vi "FitEllipse2.vi"(6 "Reject Outliers":bool, 10 "Input data":cluster{"Numeric":dbl, "Numeric":dbl}[](array[cluster])) -> (1 "XY Fit":cluster{dbl[], dbl[]}, 3 "Ellipse":T1, 5 "Valid Fit":bool)   [LabVIEW 2011]
uses:
  <vilib>/vision/NI_Vision_Development_Module.lvlib
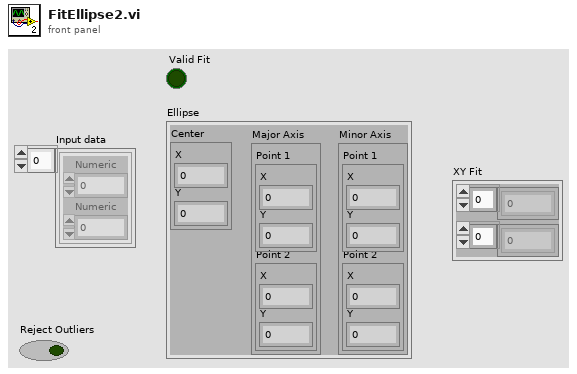
[diagram p1: front panel]
types:
  T1 = cluster{"Center":cluster{"X":sgl, "Y":sgl}, "Major Axis":cluster{"Point 1":cluster{"X":sgl, "Y":sgl}, "Point 2":cluster{"X":sgl, "Y":sgl}}, "Minor Axis":cluster{"Point 1":cluster{"X":sgl, "Y":sgl}, "Point 2":cluster{"X":sgl, "Y":sgl}}}
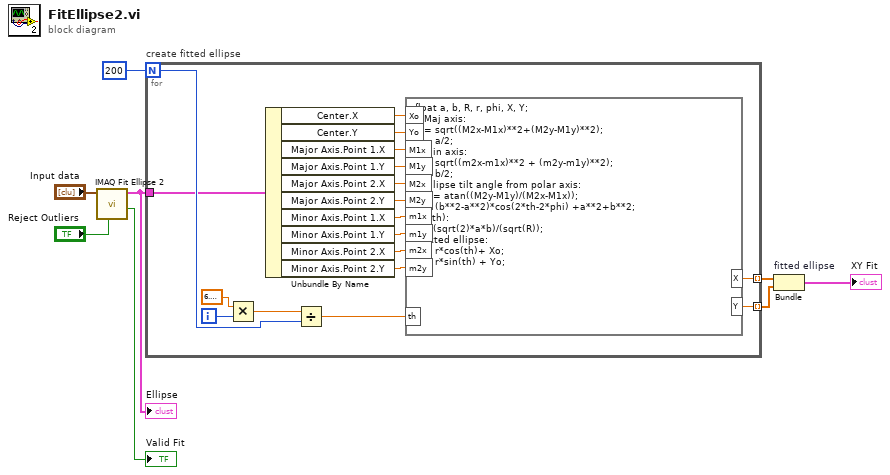
[diagram p0: block diagram]
diagram:
  n1 = call "IMAQ Fit Ellipse 2"("Reject Outliers (FALSE)"="Reject Outliers", "Radial Points"="Input data") -> ("Valid Fit"=→"Valid Fit":bool, "Ellipse"=w5:T1)  [unwired: 4 in, 4 out]
  "Ellipse" <- w5
  n2 = for "create fitted ellipse" {
    N: 200 -> [w26]
    tunnel: [w21] -> w6 mode=indexing
    tunnel: [w20] -> w7 mode=indexing
    tunnel: w5 -> [w19]
    i -> [w24]
    n3 = Multiply(x=6.283185307179586, y=w24) -> (x*y=w23:dbl)
    n4 = Unbundle By Name(w19) -> ("Center.X"=w18:sgl, "Center.Y"=w17:sgl, "Major Axis.Point 1.X"=w16:sgl, "Major Axis.Point 1.Y"=w15:sgl, "Major Axis.Point 2.X"=w14:sgl, "Major Axis.Point 2.Y"=w13:sgl, "Minor Axis.Point 1.X"=w12:sgl, "Minor Axis.Point 1.Y"=w11:sgl, "Minor Axis.Point 2.X"=w10:sgl, "Minor Axis.Point 2.Y"=w9:sgl)
    n5 = Divide(x=w23, y=w26) -> (x/y=w22:dbl)
    n6 = formula code="float a, b, R, r, phi, X, Y;\n// Maj axis:\na = sqrt((M2x-M1x)**2+(M2y-M1y)**2);\na = a/2;\n// min axis:\nb = sqrt((m2x-m1x)**2 + (m2y-m1y)**2);\nb = b/2;\n// ellipse tilt angle from polar axis:\nphi = atan((M2y-M1y)/(M2x-M1x));\nR = (b**2-a**2)*cos(2*th-2*phi) +a**2+b**2;\n// r(th):\nr = (sqrt(2)*a*b)/(sqrt(R));\n// fitted ellipse:\nX = r*cos(th)+ Xo;\nY = r*sin(th) + Yo;"("Xo"=w18, "Yo"=w17, "M1x"=w16, "M1y"=w15, "M2x"=w14, "M2y"=w13, "m1x"=w12, "m1y"=w11, "m2x"=w10, "m2y"=w9, "th"=w22) -> ("X"=w21:dbl, "Y"=w20:dbl)
  }
  n7 = Bundle "fitted ellipse"(w6, w7) -> (→"XY Fit":cluster{dbl[], dbl[]})  [unwired: 1 in]
